vi "swap.vi"(3 "index2":i32=4, 4 "index1":i32=3, 5 "Array_in":T1(array[cluster])) -> (2 "Array_out":T1(array[cluster]))   [LabVIEW 2011]
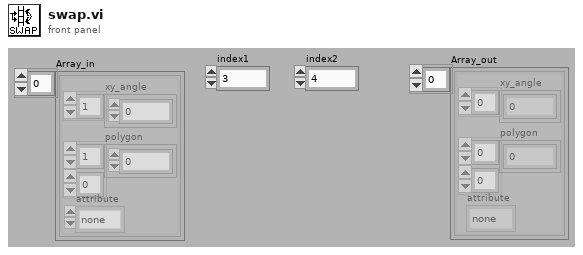
[diagram p1: front panel]
types:
  T1 = cluster{"xy_angle":dbl[], "polygon":dbl[][], "attribute":enum16{"none", "transparent", "reflective", "white", "black", "red", "yellow", "green", "blue", "pink"}}[]
  T2 = cluster{"xy_angle":dbl[], "polygon":dbl[][], "attribute":enum16{"none", "transparent", "reflective", "white", "black", "red", "yellow", "green", "blue", "pink"}}
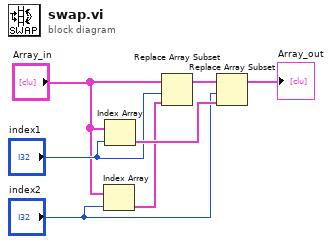
[diagram p0: block diagram]
diagram:
  n1 = Index Array(array="Array_in", index="index2") -> (element=w6:T2)
  n2 = Index Array(array="Array_in", index="index1") -> (element=w7:T2)
  n3 = Replace Array Subset(array="Array_in", new element=w6, index="index1") -> (w2:T1)
  n4 = Replace Array Subset(array=w2, new element=w7, index="index2") -> (→"Array_out":T1)
